vi "Estimate Test Coverage.vi"(8 "error in (no error)":errorcluster, 9 "Scan Options":T1={"Ignore vi.lib"=TRUE, "Ignore user.lib"=TRUE, "Ignore private methods"=FALSE, "Ignore non VIs"=TRUE, "Shallow scan (FALSE)"=FALSE}, 10 "Test Path (Tests folder -- including _framework)":path, 11 "Source Path (lvproj, lvclass, vi)":path) -> (0 "error out":errorcluster, 1 "Coverage Results":T2 {"% Coverage" format="%.1f"}, 2 "VIs Without Test Coverage by path":path[](array[path]))   [LabVIEW 2009, in "GraphicalTestRunner.lvlib"]
uses:
  GraphicalTestRunner.lvlib
  EstimationResults--Cluster.ctl
  ScanOptions--Cluster.ctl
  <userlib>/_OpenG.lib/array/array.llb/Conditional Auto-Indexing Tunnel (Path)__ogtk.vi
  <userlib>/_OpenG.lib/array/array.llb/Filter 1D Array (Path)__ogtk.vi
  <userlib>/_OpenG.lib/array/array.llb/Remove Duplicates from 1D Array (Path)__ogtk.vi
  <userlib>/_OpenG.lib/file/file.llb/Strip Path Extension - Path__ogtk.vi
  Libraries/VITesterUtilities.lvlib
panel:
  out "VIs Without Test Coverage":string[](array[string])
  # "Copyright © 2007 James Kring, Inc. All rights reserved.\n\nAuthor: Omar Mussa [omar.mussa@jameskring.com]\n\nThis library is provided \"AS IS\" ,WITHOUT WARRANTIES OR \nCONDITIONS OF ANY KIND, either express or implied.\n\nJames Kring, Inc. -- http://www.jameskring.com"
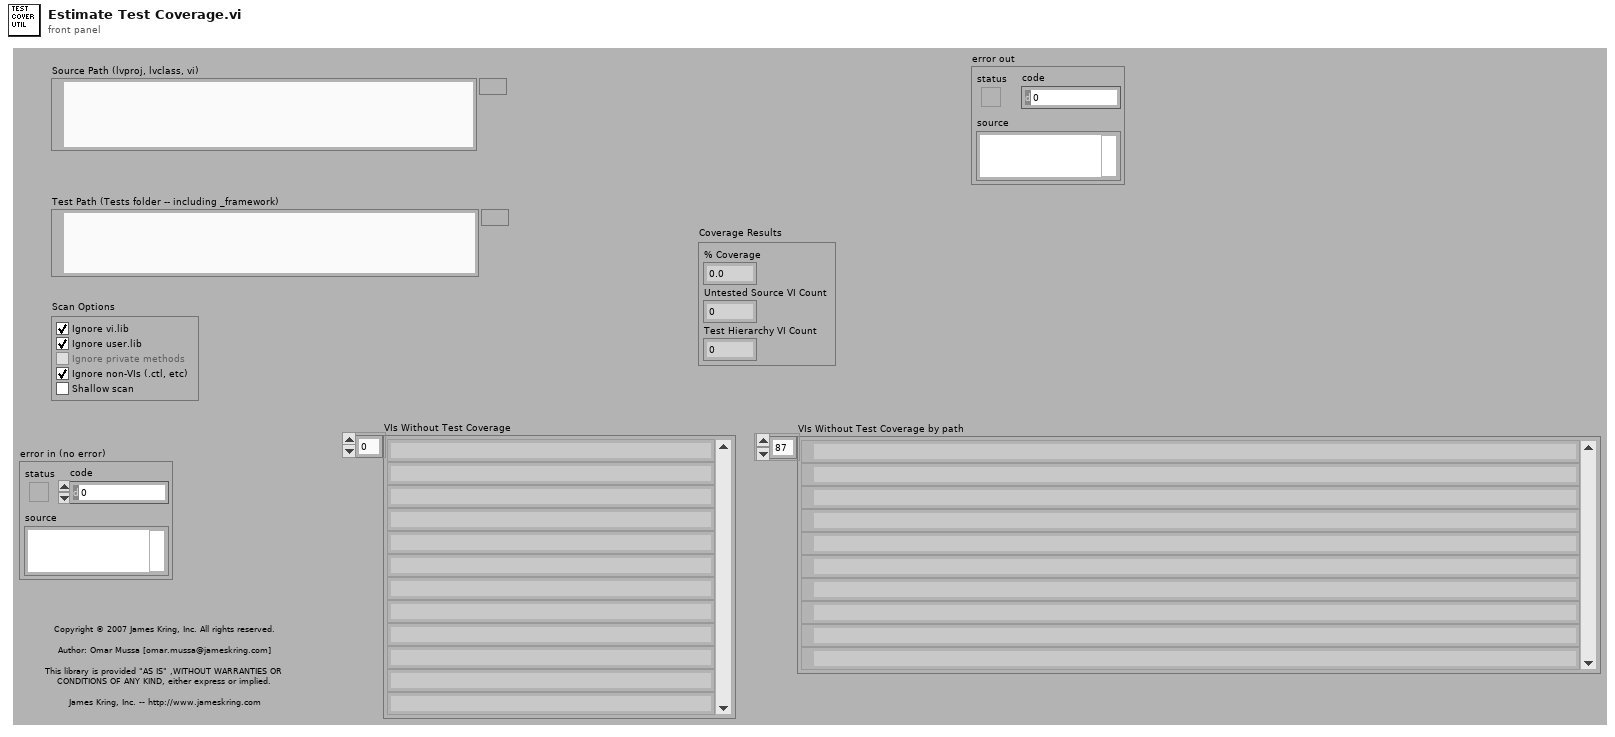
[diagram p1: front panel]
types:
  T1 = typedef "GraphicalTestRunner.lvlib/ScanOptions--Cluster.ctl" = cluster{"Ignore vi.lib":bool, "Ignore user.lib":bool, "Ignore private methods":bool, "Ignore non VIs":bool, "Shallow scan (FALSE)":bool}
  T2 = typedef "GraphicalTestRunner.lvlib/EstimationResults--Cluster.ctl" = cluster{"% Coverage":dbl, "Untested Source VI Count":i32, "Test Hierarchy VI Count":i32}
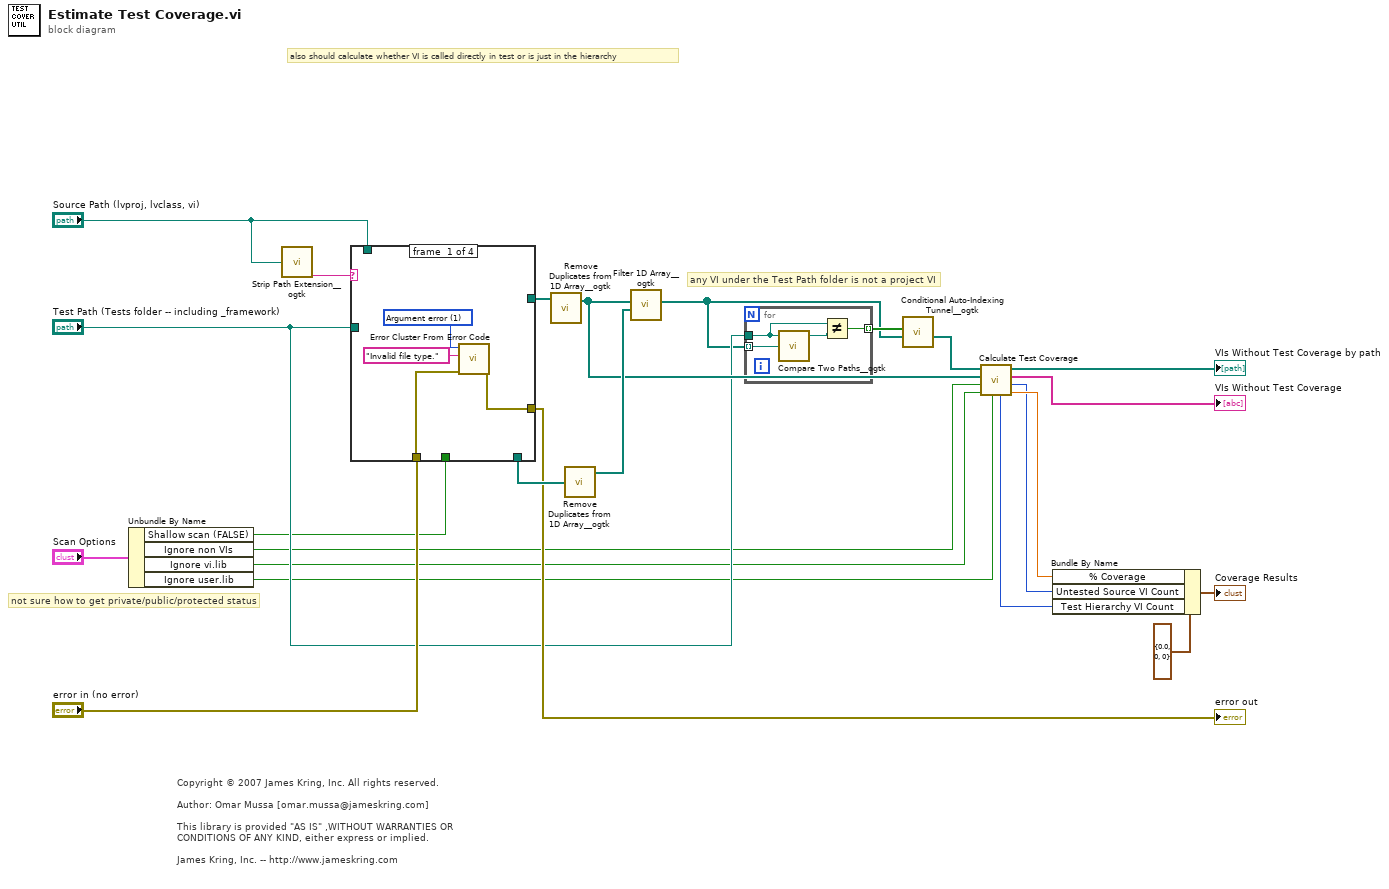
[diagram p0: block diagram]
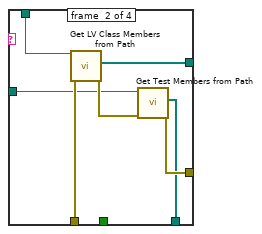
[diagram p2: hidden frame]
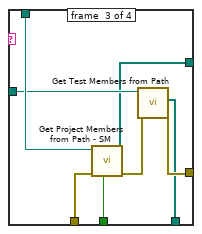
[diagram p3: hidden frame]
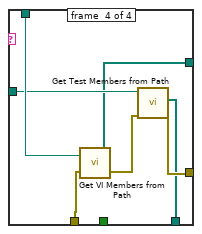
[diagram p4: hidden frame]
diagram:
  # "any VI under the Test Path folder is not a project VI"
  # "Copyright © 2007 James Kring, Inc. All rights reserved.\n\nAuthor: Omar Mussa [omar.mussa@jameskring.com]\n\nThis library is provided \"AS IS\" ,WITHOUT WARRANTIES OR \nCONDITIONS OF ANY KIND, either express or implied.\n\nJames Kring, Inc. -- http://www.jameskring.com"
  # "also should calculate whether VI is called directly in test or is just in the hierarchy"
  # "not sure how to get private/public/protected status"
  n1 = Unbundle By Name("Scan Options") -> ("Shallow scan (FALSE)"=w4:bool, "Ignore non VIs"=w3:bool, "Ignore vi.lib"=w2:bool, "Ignore user.lib"=w1:bool)
  n2 = call-poly <userlib>:"Strip Path Extension__ogtk.vi"("path"="Source Path (lvproj, lvclass, vi)") -> ("extension"=w19:string)  [unwired: 1 out]
  n3 = case shown="\"lvproj\"" w19 {
    tunnel: "Test Path (Tests folder -- including _framework)" -> [_ w30 w39 w46]
    tunnel: [_ w29 w37 w44] -> w24
    tunnel: [_ w33 w38 w45] -> w17
    tunnel: "error in (no error)" -> [w28 w35 w43 w50]
    tunnel: [w27 w31 w40 w47] -> w21
    tunnel: "Source Path (lvproj, lvclass, vi)" -> [_ w34 w42 w49]
    tunnel: w4 -> [_ _ w36 _]
    frame #0 {
      w25 = 1 items=["No error", "Argument error", "Memory is full", "Out of zone", "End of file", "File already open", "Generic file I/O error", "File not found", "File permission error", "Disk is full", "Duplicate path", "Too many files open", "System feature not enabled", "Resource file not found", "Cannot add resource", "Resource not found", "Image not found", "Image memory error", "Pen does not exist", "Config type invalid", "Config token not found", "Config parse error", "Config memory error", "Bad external code format", "Bad external code offset", "External code not present", "Null window", "Destroy window error", "Null menu", "Print aborted", "Bad print record", "Print driver error", "Windows error during printing", "Memory error during printing", "Print dialog error", "Generic print error", "Invalid device refnum", "Device not found", "Device parameter error", "Device unit error", "Cannot open device", "Device call aborted", "Generic error", "Cancelled by user", "Object ID too low", "Object ID too high", "Object not in heap", "Unknown heap", "Unknown object (invalid DefProc)", "Unknown object (DefProc not in table)", "Message out of range", "Invalid (null) method", "Unknown message", "Manager call not supported", "Bad address", "Network operation in progress", "Network operation timed out", "Connection is busy", "Network attribute not supported", "Network error", "Address in use", "System out of memory", "Connection aborted", "Connection refused", "Not connected", "Already connected", "Connection closed", "Initialization error (interapplication manager)", "Bad occurrence", "Wait on unbound occurrence handler", "Occurrence queue overflow", "Datalog type conflict", "Unused", "Unrecognized type (interapplication manager)", "Memory corrupt", "Failed to make temporary DLL", "Old CIN version", "Drag socket not found", "Failed to load drop-object", "Failed to register OLE object", "Failed to release OLE object", "Format specifier type mismatch", "Unknown format specifier", "Too few format specifiers", "Too many format specifiers", "Scan failed", "Newer CIN version", "Error converting to variant", "Runtime menu error", "Password tampered", "Variant attribute not found", "Incompatible variant data type", "Event data is not available", "Event Store is not present", "Occurrence is not found", "Event Queue is not created", "Event info is not available", "Refnum passed is NULL", "Error retrieving Class GUID", "Error retrieving CoClass GUID", "Error retrieving TypeLib GUID.", "Bad built application magic bytes.", "Specific driver is different from the specific driver associated with the Logical Name.", "There is no session opened to the class driver.", "Max Error", "MAX - Error with config objects", "MAX - Error loading configuration", "MAX - Group not supported"]
      n4 = call <vilib>:"Error Cluster From Error Code.vi"("error in (no error)"=w28, "error message (\"\")"="Invalid file type." ("error message (\"\")"), "error code (0)"=w25) -> ("error out"=w27:errorcluster)  [unwired: 6 in]
    }
    frame #1 {
      n5 = call "Get LV Class Members from Path.vi"("error in (no error)"=w35, "Class Path"=w34) -> ("error out"=w32:errorcluster, "LV Class Members"=w33:path[])  [unwired: 8 in]
      n6 = call "Get Test Members from Path.vi"("error in (no error)"=w32, "Tests Path"=w30) -> ("error out"=w31:errorcluster, "Test Members"=w29:path[])  [unwired: 8 in]
    }
    frame #2 {
      n7 = call "Get Project Members from Path - SM.vi"("Shallow Scan"=w36, "error in"=w43, "Project Path"=w42) -> ("error out"=w41:errorcluster, "Project Members"=w38:path[])  [unwired: 7 in]
      n8 = call "Get Test Members from Path.vi"("error in (no error)"=w41, "Tests Path"=w39) -> ("error out"=w40:errorcluster, "Test Members"=w37:path[])  [unwired: 8 in]
    }
    frame #3 {
      n9 = call "Get VI Members from Path.vi"("error in (no error)"=w50, "VI Path"=w49) -> ("error out"=w48:errorcluster, "VI Members"=w45:path[])
      n10 = call "Get Test Members from Path.vi"("error in (no error)"=w48, "Tests Path"=w46) -> ("error out"=w47:errorcluster, "Test Members"=w44:path[])  [unwired: 8 in]
    }
  }
  "error out" <- w21
  n11 = call-poly <userlib>:"Remove Duplicates from 1D Array__ogtk.vi"("Input Array"=w17) -> ("Output Array"=w18:path[])  [unwired: 1 out]
  n12 = call-poly <userlib>:"Remove Duplicates from 1D Array__ogtk.vi"("Input Array"=w24) -> ("Output Array"=w23:path[])  [unwired: 1 out]
  n13 = call-poly <userlib>:"Filter 1D Array__ogtk.vi"("items to filter"=w23, "array"=w18) -> ("filtered array"=w12:path[])  [unwired: 4 in, 1 out]
  n14 = for {
    tunnel: w12 -> [w54] mode=indexing
    tunnel: "Test Path (Tests folder -- including _framework)" -> [w52]
    tunnel: [w51] -> w13 mode=indexing
    n15 = call <userlib>:"Compare Two Paths__ogtk.vi"("path2"=w54, "path1"=w52) -> ("common path"=w53:path)  [unwired: 1 in, 2 out]
    n16 = Not Equal?(x=w52, y=w53) -> (x != y?=w51:bool)
  }
  n17 = call-poly <userlib>:"Conditional Auto-Indexing Tunnel__ogtk.vi"("Array in"=w12, "Elements to keep"=w13) -> ("Filtered Array out"=w11:path[])  [unwired: 5 in]
  n18 = call "Calculate Test Coverage.vi"("Ignore user.lib"=w1, "Ignore vi.lib"=w2, "Ignore non VIs"=w3, "Test Members"=w18, "Project Members"=w11) -> ("% Coverage"=w9:dbl, "Unused VI Count"=w8:i32, "VI Names without coverage"=→"VIs Without Test Coverage":string[], "VIs without coverage"=→"VIs Without Test Coverage by path":path[], "Test VI Count"=w7:i32)  [unwired: 2 in]
  n19 = Bundle By Name(cluster=T2 {"% Coverage"=0.0, "Untested Source VI Count"=0, "Test Hierarchy VI Count"=0} ("Results"), "% Coverage"=w9, "Untested Source VI Count"=w8, "Test Hierarchy VI Count"=w7) -> (→"Coverage Results":T2)
